vi "Simple Read.vi"(4 "Abs_String in":refnum<class "Abs_String.lvclass">) -> (1 "String":string)   [LabVIEW 2021, in "Abs_String.lvclass"]
uses:
  Abs_String.lvclass
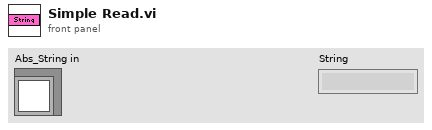
[diagram p1: front panel]
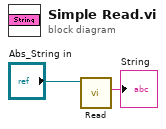
[diagram p0: block diagram]
diagram:
  n1 = call-dynamic "Read.vi"("Abs_String in"="Abs_String in") -> ("String"=→"String":string)  [unwired: 8 in, 2 out]
